vi "RSNRPZ Get S-Parameter Device List.vi"(8 "error in (no error)":errorcluster, 9 "Buffer Size (1000)":i32=1000, 10 "Channel (1)":i32=1 format="%.0g", 11 "VISA session":refnum<visa-resource-name> caption="VISA resource name") -> (0 "error out":errorcluster, 2 "S-Parameter Device List":string, 3 "dup VISA session":refnum<visa-resource-name> caption="VISA resource name")   [LabVIEW 2010]
doc: "This VI gets list of S-Parameter devices. \n\nNote(s):\n\n(1) This VI is available only on NRP-Z81.\n\nRemote-control command(s):\nSENS:CORR:SPD:LIST?"
uses:
  rsnrpz_32.dll
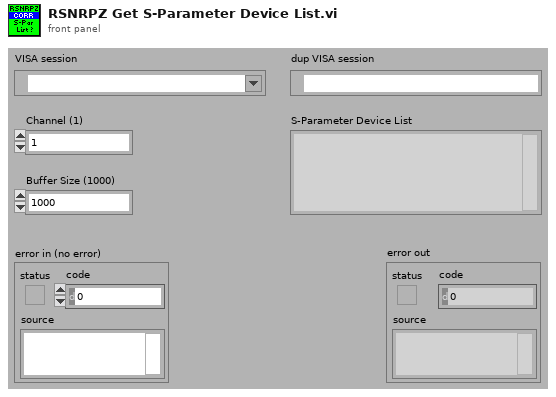
[diagram p1: front panel]
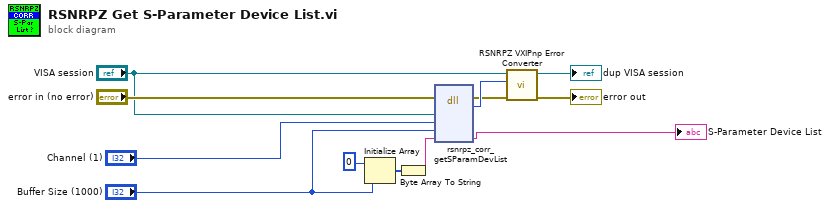
[diagram p0: block diagram]
diagram:
  n1 = Initialize Array(u8 0 ("element"), "Buffer Size (1000)") -> (w7:u8[])
  n2 = Byte Array To String(unsigned byte array=w7) -> (string=w8:string)
  n3 = dll-call lib="rsnrpz_32.dll" fn="rsnrpz_corr_getSParamDevList"(error in="error in (no error)", "Instrument Handle"="VISA session", "Channel"="Channel (1)", "Buffer Size"="Buffer Size (1000)", "S-Parameter Device List"=w8) -> (error out=w5:errorcluster, "return type"=w9:i32, "S-Parameter Device List"=→"S-Parameter Device List":string)  [unwired: 5 in, 1 out]
  n4 = call <instrlib>:"RSNRPZ VXIPnp Error Converter.vi"("error in"=w5, "VXIPnp error code"=w9, "VISA session"="VISA session") -> ("error out"=→"error out":errorcluster, "dup VISA session"=→"dup VISA session":refnum<visa-resource-name>)  [unwired: 7 in]
